vi "PI_Image_Scanner_Prepare_Dlg.vi"(0 "System no.":i32, 1 "Picture Size":dbl[](array[numeric]), 2 "Pixels":u16[](array[numeric]), 5 "Axis":enum32{"x-y", "x-z", "y-z"}(ring), 7 "Scanner Divider":i32, 11 "error in":errorcluster, 12 "Learning loop":bool=TRUE) -> (4 "System no. (dup)":i32, 8 "Measurement time [s]":i32, 15 "error out":errorcluster)   [LabVIEW 8.6]
panel:
  out "Programming scanner":u8(slide) caption="Preparing Scanner" scale=0.0..100.0
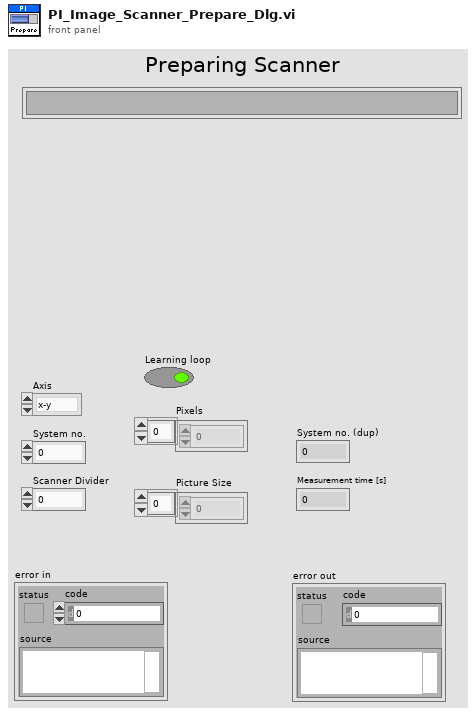
[diagram p1: front panel]
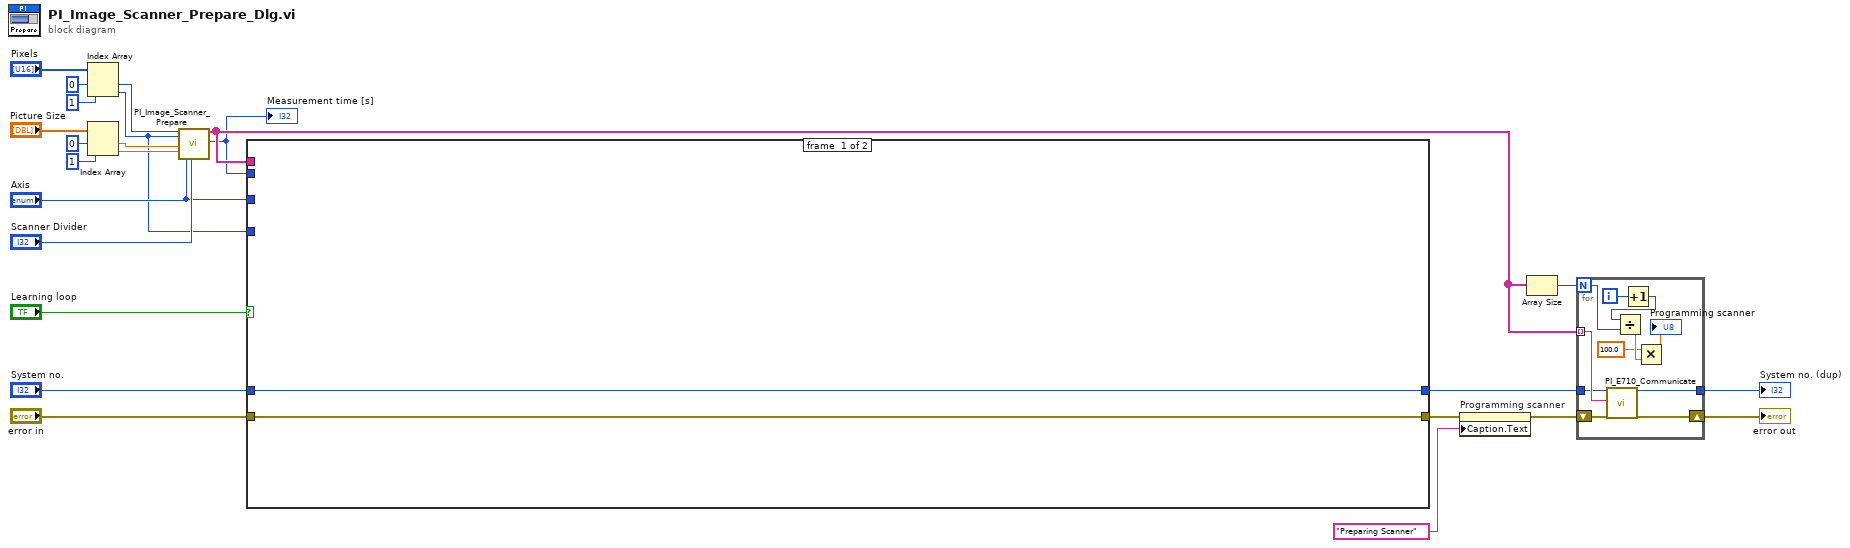
[diagram p0: block diagram]
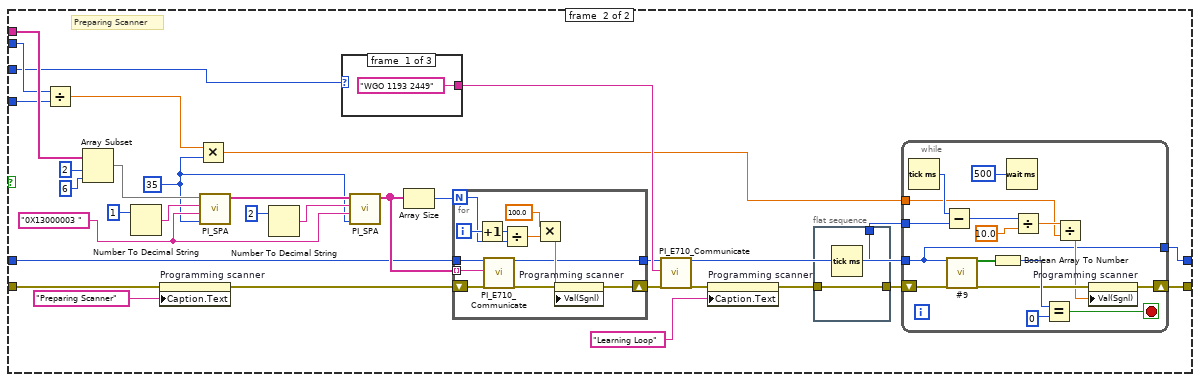
[diagram p2: hidden frame]
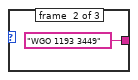
[diagram p3: hidden frame]
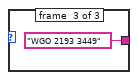
[diagram p4: hidden frame]
diagram:
  n1 = Index Array(array="Pixels", index #1=0 ("index"), index #2=1 ("index")) -> (element #1=w12:u16, element #2=w6:u16)
  n2 = Index Array(array="Picture Size", index #1=0 ("index"), index #2=1 ("index")) -> (element #1=w17:dbl, element #2=w16:dbl)
  n3 = call "PI_Image_Scanner_Prepare.vi"("x-Pixel"=w12, "y-Pixel"=w6, "Picture size x"=w17, "Picture size y"=w16, "Axis"="Axis", "Scanner Divider"="Scanner Divider") -> ("Commandset out"=w9:string[], "Measurement time / [s]"=w7:i32)  [unwired: 12 in]
  "Measurement time [s]" <- w7
  n4 = case shown="True" "Learning loop" {
    tunnel: w9 -> [_ w58]
    tunnel: w7 -> [_ w42]
    tunnel: "Axis" -> [_ w35]
    tunnel: w6 -> [_ w34]
    tunnel: "System no." -> [w25 w33]
    tunnel: "error in" -> [w26 w32]
    tunnel: [w26 w28] -> w3
    tunnel: [w25 w27] -> w1
    frame #0 {
    }
    frame #1 {
      w43 = u16 35 ("Value")
      w49 = "0X13000003 " ("string")
      # "Preparing Scanner"
      n5 = Divide(x=w42, y=w34) -> (x/y=w44:dbl)
      n6 = Array Subset(array=w58, index=2 ("Index"), length=6 ("Länge")) -> (w55:string[])
      n7 = Number To Decimal String(number=1 ("Wert")) -> (decimal integer string=w52:string)  [unwired: 1 out]
      n8 = property on="Programming scanner" class="Slide (strict)"(error in=w32, "Caption.Text"="Preparing Scanner" ("Beschriftung.Text")) -> (error out=w39:errorcluster)  [unwired: 1 in, 1 out]
      n9 = Multiply(x=w44, y=w43) -> (x*y=w41:dbl)
      n10 = call "PI_SPA.vi"("Value"=w43, "Register"=w49, "Axis"=w52, "Commandset in"=w55) -> ("Commandset out"=w53:string[])  [unwired: 7 out]
      n11 = Number To Decimal String(number=2 ("Wert")) -> (decimal integer string=w50:string)  [unwired: 1 out]
      n12 = case shown="\"x-y\", Default" w35 {
        tunnel: ["WGO 1193 2449" ("String to send") "WGO 1193 3449" ("String to send") "WGO 2193 3449" ("String to send")] -> w48
        frame #0 {
        }
        frame #1 {
        }
        frame #2 {
        }
      }
      n13 = call "PI_SPA.vi"("Value"=w43, "Register"=w49, "Axis"=w50, "Commandset in"=w53) -> ("Commandset out"=w47:string[])  [unwired: 7 out]
      n14 = Array Size(array=w47) -> (size(s)=w46:i32)
      n15 = for {
        N: w46 -> [w89]
        tunnel: w47 -> [w92] mode=indexing
        tunnel: [w85] -> w45
        shift-right: [w82] -> w59
        shift-left: w39 -> [w84]
        tunnel: w33 -> [w81]
        i -> [w91]
        n16 = Increment(x=w91) -> (x+1=w90:i32)
        n17 = call "PI_E710_Communicate.vi"("System no."=w81, "String to send"=w92, "error in"=w84) -> ("System no. (dup)"=w85:i32, "error out"=w83:errorcluster)  [unwired: 14 in, 1 out]
        n18 = Divide(x=w90, y=w89) -> (x/y=w88:dbl)
        n19 = Multiply(x=100.0, y=w88) -> (x*y=w86:dbl)
        n20 = property on="Programming scanner" class="Slide (strict)"(error in=w83, "Val(Sgnl)"=w86) -> (error out=w82:errorcluster)  [unwired: 1 in, 1 out]
      }
      n21 = call "PI_E710_Communicate.vi"("System no."=w45, "String to send"=w48, "error in"=w59) -> ("System no. (dup)"=w36:i32, "error out"=w38:errorcluster)  [unwired: 14 in, 1 out]
      n22 = property on="Programming scanner" class="Slide (strict)"(error in=w38, "Caption.Text"="Learning Loop" ("Beschriftung.Text")) -> (error out=w31:errorcluster)  [unwired: 1 in, 1 out]
      n23 = flat-sequence {
        tunnel: w31 -> [w61]
        tunnel: [w61] -> w30
        tunnel: [w60] -> w29
        frame #0 {
          n24 = Tick Count (ms)() -> (millisecond timer value=w60:u32)
        }
      }
      n25 = while {
        tunnel: w36 -> [w62]
        tunnel: w41 -> [w71]
        tunnel: w29 -> [w72]
        shift-right: [w63] -> w28
        shift-left: w30 -> [w70]
        tunnel: [w62] -> w27
        stop <- w66 stop-if-true
        n26 = Tick Count (ms)() -> (millisecond timer value=w76:u32)
        n27 = Subtract(x=w76, y=w72) -> (x-y=w75:u32)
        n28 = call "#9.vi"("System no."=w62, "error in"=w70) -> ("WG running?"=w69:bool[], "error out"=w65:errorcluster)  [unwired: 16 in]
        n29 = Boolean Array To Number(Boolean array=w69) -> (number=w68:u32)
        n30 = Wait (ms)(milliseconds to wait=u32 500 ("Zu wartende ms")) -> ()  [unwired: 1 out]
        n31 = Divide(x=w75, y=10.0) -> (x/y=w73:dbl)
        n32 = Equal?(x=w68, y=u32 0) -> (x = y?=w66:bool)
        n33 = Divide(x=w73, y=w71) -> (x/y=w64:dbl)
        n34 = property on="Programming scanner" class="Slide (strict)"(error in=w65, "Val(Sgnl)"=w64) -> (error out=w63:errorcluster)  [unwired: 1 in, 1 out]
      }
    }
  }
  n35 = property on="Programming scanner" class="Slide (strict)"(error in=w3, "Caption.Text"="Preparing Scanner" ("Label.Text")) -> (error out=w11:errorcluster)  [unwired: 1 in, 1 out]
  n36 = Array Size(array=w9) -> (size(s)=w21:i32)
  n37 = for {
    N: w21 -> [w101]
    tunnel: w9 -> [w97] mode=indexing
    shift-right: [w95] -> w23
    shift-left: w11 -> [w96]
    tunnel: w1 -> [w94]
    tunnel: [w93] -> w22
    i -> [w103]
    n38 = call "PI_E710_Communicate.vi"("System no."=w94, "String to send"=w97, "error in"=w96) -> ("System no. (dup)"=w93:i32, "error out"=w95:errorcluster)  [unwired: 14 in, 1 out]
    n39 = Increment(x=w103) -> (x+1=w102:i32)
    n40 = Divide(x=w102, y=w101) -> (x/y=w100:dbl)
    n41 = Multiply(x=100.0, y=w100) -> (x*y=→"Programming scanner":dbl)
  }
  "error out" <- w23
  "System no. (dup)" <- w22
